vi "Go To Annoucing.vi"(8 "error in (no error)":errorcluster, 11 "Executing State in":refnum<class "Executing State.lvclass">) -> (0 "error out":errorcluster, 3 "State out":refnum<class "State Actor.lvclass">)   [LabVIEW 2013, in "Receiver.lvlib" / "Commands.lvlib" / "Connect.lvlib" / "Executing States.lvlib" / "Executing State.lvclass"]
uses:
  Executing State.lvclass
  <vilib>/ni/Actors/State Actor/State Actor/State Actor.lvclass
  Annoucing/Annoucing.lvclass
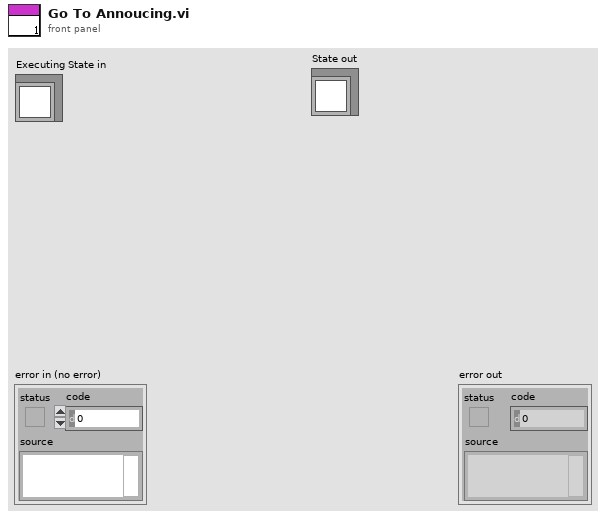
[diagram p1: front panel]
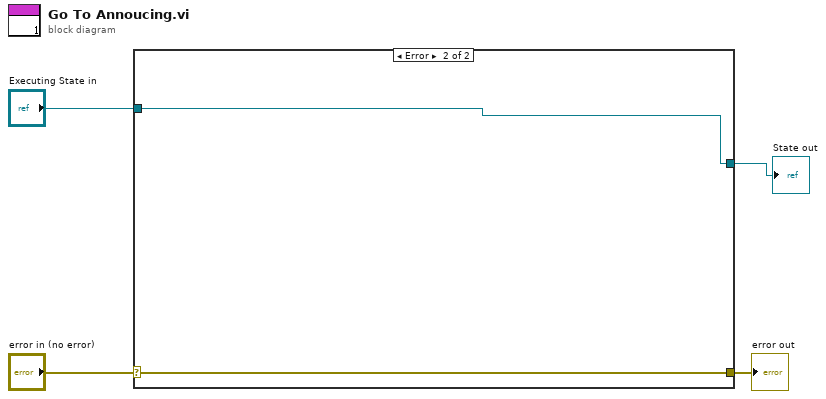
[diagram p0: block diagram]
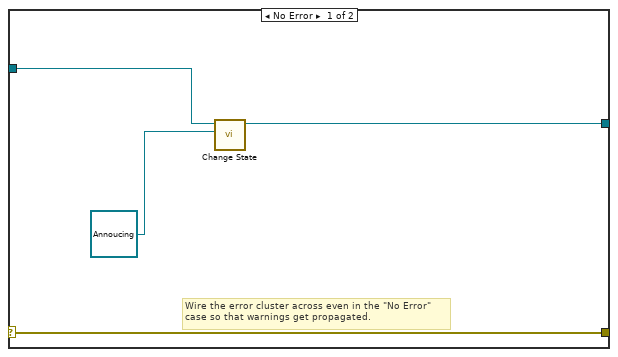
[diagram p2: hidden frame]
diagram:
  n1 = case shown="Error" "error in (no error)" {
    selector: "error in (no error)" -> [w8 w10]
    tunnel: [w8 w10] -> w3
    tunnel: "Executing State in" -> [w7 w9]
    tunnel: [w5 w9] -> w1
    frame No Error {
      # "Wire the error cluster across even in the \"No Error\"\ncase so that warnings get propagated."
      n2 = call <vilib>:"Change State.vi"("New State in"=refnum<class "Annoucing.lvclass"> refnum ("Receiver.lvlib:Commands.lvlib:Connect.lvlib:Executing States.lvlib:Annoucing.lvclass"), "State in"=w7) -> ("State out"=w5:refnum<class "State Actor.lvclass">)  [unwired: 8 in, 1 out]
    }
    frame Error {
    }
  }
  "error out" <- w3
  "State out" <- w1
